vi "ReadFromFIFO.vi"() -> (2 "This is what I told you!":string)   [LabVIEW 2011]
doc: "Elizabeth Mahon\nNot finished yet\nBased off of example from LabView and IGVC 3.2.1 Read VectorNav.\n\nDoesn't take in anything, gives string result.\n\nNot sure what folder this should be in..."
uses:
  <vilib>/FPGAPlugInAG/cRIO-9113/niLvFpga_Open_cRIO-9113.vi
  <vilib>/rvi/interface/common/dynamic/niFpgaDynamicAddResources.vi
  <vilib>/Utility/error.llb/Error Cluster From Error Code.vi
  <vilib>/rvi/errors/niLvFpgaAdjustHostInterfaceError.vi
  <vilib>/rvi/interface/nirviOpenFPGA/nirviOpenFPGA.xnode
  FPGA Bitfiles/SailBot_FPGATarget_WriteToFIFO_EBA82491.lvbitx
  1A-FPGA/1A Code/WriteToFIFO.vi
  <vilib>/rvi/interface/nirviMethod/nirviMethod.xnode
  <vilib>/FPGAPlugInAG/Dynamic/niLvFpga_ReadFifo_Dynamic.vi
  <vilib>/rvi/errors/niLvFpgaMergeErrorWithErrorCode.vi
panel:
  out "Status Out":enum16{"Reading", "Time Out!"}(ring)
  out "Data":i16[](array[numeric])
  out "Elements Remaining":u32
  in  "stop":bool
  in  "Status":enum16{"Reading", "Time Out!"}(ring)
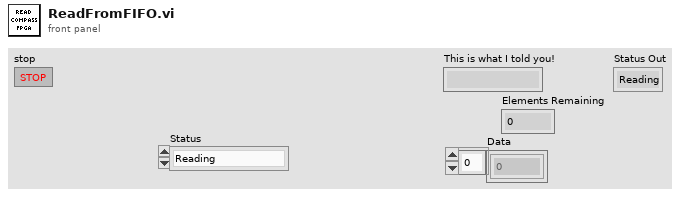
[diagram p1: front panel]
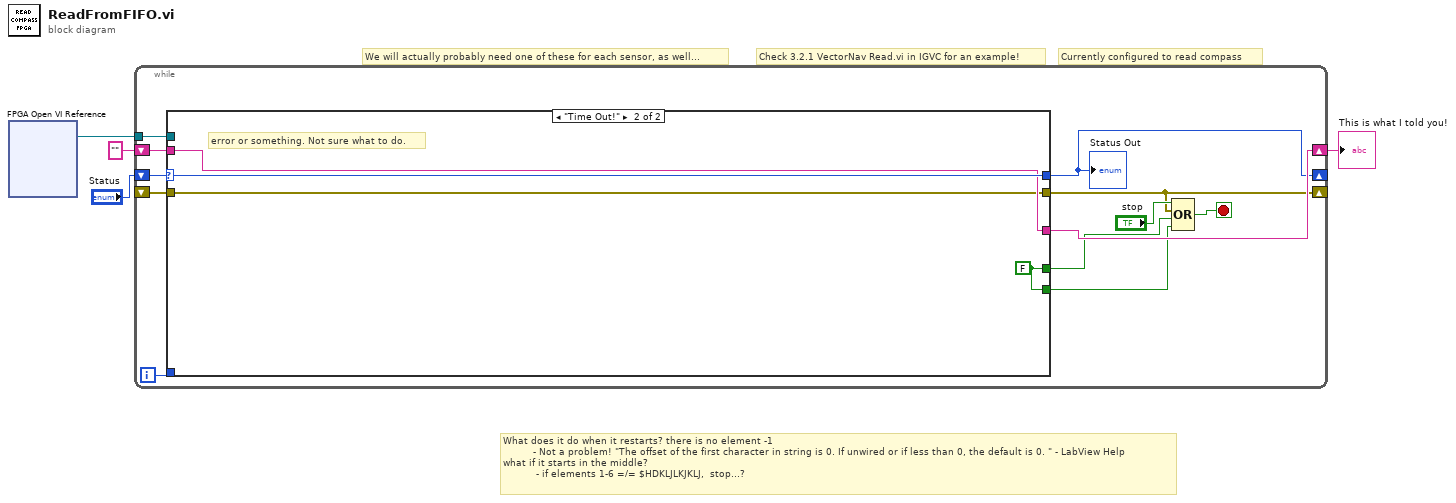
[diagram p0: block diagram]
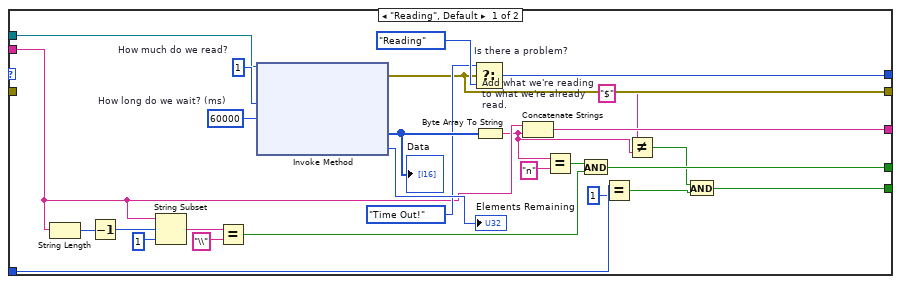
[diagram p2: hidden frame]
diagram:
  # "What does it do when it restarts? there is no element -1\n          - Not a problem! \"The offset of the first character in string is 0. If unwired or if less than 0, the default is 0. \" - LabView Help\nwhat if it starts in the middle?\n           - if elements 1-6 =/= $HDKLJLKJKLJ,  stop...?"
  # "Currently configured to read compass"
  # "Check 3.2.1 VectorNav Read.vi in IGVC for an example!"
  # "We will actually probably need one of these for each sensor, as well..."
  n1 = xnode "FPGA Open VI Reference"() -> ("FPGA VI Reference Out"=w4:refnum<k20>)  [unwired: 2 in, 1 out]
  n2 = while {
    tunnel: w4 -> [w16]
    shift-right: [w14] -> w3
    shift-left: "" -> [w15]
    shift-right: [w12] -> _
    shift-left: "Status" -> [w13]
    shift-right: [w9] -> _
    shift-left: _ -> [w8]
    i -> [w6]
    stop <- w10 stop-if-true
    n3 = case shown="\"Time Out!\"" w13 {
      selector: w13 -> [_ w47]
      tunnel: w16 -> [w41 _]
      tunnel: w15 -> [w24 w46]
      tunnel: [w34 w46] -> w14
      tunnel: [w39 w47] -> w12
      tunnel: [w35 w45] -> w9
      tunnel: w8 -> [_ w45]
      tunnel: [w25 w44] -> w7
      tunnel: w6 -> [w21 _]
      tunnel: [w17 w44] -> w5
      frame "Reading", Default {
        w42 = 60000  # How long do we wait? (ms)
        w43 = u32 1  # How much do we read?
        n4 = String Length(string=w24) -> (length=w32:i32)
        n5 = Decrement(x=w32) -> (x-1=w31:i32)
        n6 = String Subset(string=w24, offset (0)=w31, length (rest)=1 ("length (rest)")) -> (substring=w29:string)
        n7 = Equal?(x=w29, y="\\") -> (x = y?=w26:bool)
        n8 = xnode "Invoke Method"("FPGA VI Reference In"=w41, "Number of Elements"=w43, "Timeout (ms)"=w42) -> ("error out"=w35:errorcluster, "Data"=w40:i16[], "Elements Remaining"=→"Elements Remaining":u32)  [unwired: 1 in, 1 out]
        "Data" <- w40
        n9 = Select "Is there a problem?"(t=enum16{"Reading", "Time Out!"}."Time Out!", s=w35, f=enum16{"Reading", "Time Out!"}."Reading" ("Status 2")) -> (s? t:f=w39:enum16{"Reading", "Time Out!"})
        n10 = Byte Array To String(unsigned byte array=w40) -> (string=w23:string)
        n11 = Concatenate Strings "Add what we're reading to what we're already read."(w24, w23) -> (w34:string)
        n12 = Equal?(x=w23, y="n") -> (x = y?=w27:bool)
        n13 = And(x=w27, y=w26) -> (x .and. y?=w25:bool)
        n14 = Equal?(x=w21, y=1) -> (x = y?=w19:bool)
        n15 = Not Equal?(x="$", y=w23) -> (x != y?=w18:bool)
        n16 = And(x=w18, y=w19) -> (x .and. y?=w17:bool)
      }
      frame "Time Out!" {
        w44 = FALSE
        # "error or something. Not sure what to do."
      }
    }
    "Status Out" <- w12
    n17 = Compound Arithmetic op=OR("stop", w9, w7, w5) -> (w10:bool)
  }
  "This is what I told you!" <- w3
